vi "TestExec.Run Executable.vi"(6 "Reset":bool, 7 "Vars":variant, 8 "error in":errorcluster, 9 "Timeout(s)":dbl=500.0 caption="Time Out(s)" format="%.2f", 10 "Output Folder":path, 11 "Utility Config File":path) -> (0 "Error":errorcluster, 3 "RTN Data":T1 {"MeasData"."Status" items=["LOG", "PASS", "FAIL", "ERROR"]; "Attr"."Status" items=["LOG", "PASS", "FAIL", "ERROR"]; "Num"."Status" items=["LOG", "PASS", "FAIL", "ERROR"]})   [LabVIEW 2024]
uses:
  TestExec.Local Result Data.ctl
  Results/Result.Attribute.ctl
  Results/Result.Measurement and Attribute Item Status.ctl
  Results/Result.Numeric.ctl
  Results/Result.Limit Type.ctl
  Results/Result XML/TestResult.SW Item.ctl
  Reports/Report.Result FileDataObject.ctl
  Results/Result.Measurement Item.ctl
  Cmd Exe/CmdExe.Setup Params.ctl
  Cmd Exe/CmdExe.Output Error Check Setup.ctl
  <vilib>/Utility/error.llb/Trim Whitespace One-Sided.vi
  Errors.lvlib
  <vilib>/KATE/Time/Time Utils.lvlib
panel:
  in  "Tab Control":enum32{"Execute", "Results"}(tab)
  out "Active":bool
  out "Sys Exec Commands":string
  out "Sys Exec STDOut":string
  out "Dur(s)":dbl caption="Duration(s)" format="%.3f"
  out "Rslt":u32(colorbox)=13816530 caption="Exe"
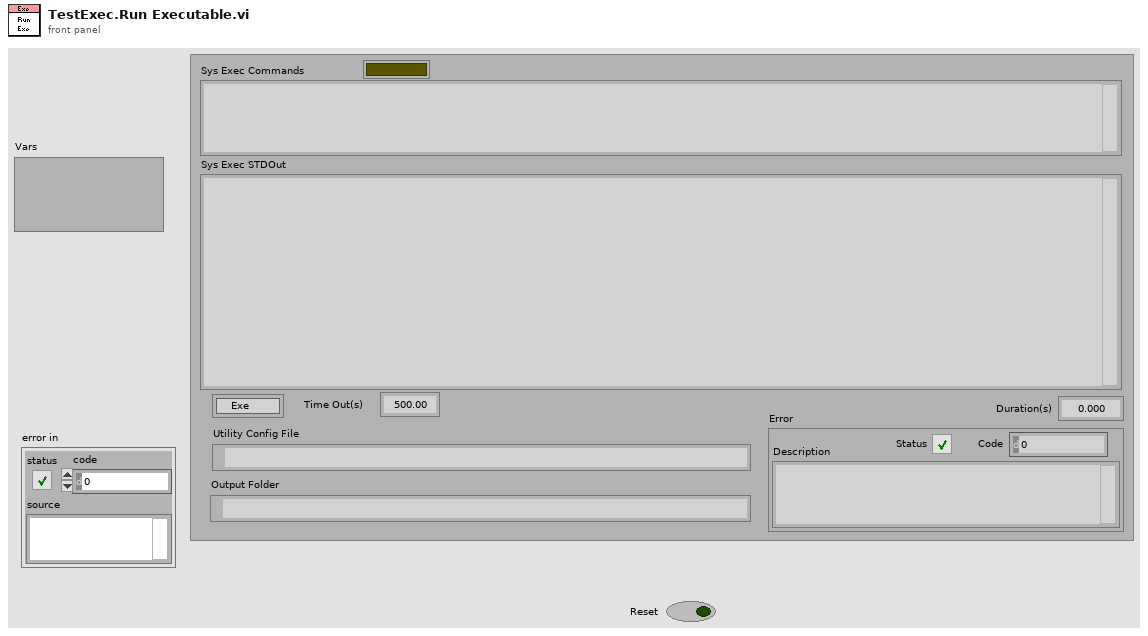
[diagram p1: front panel]
types:
  T1 = typedef "TestExec.Local Result Data.ctl" = cluster{"Attr":T2[], "Num":T4[], "UUT Props":string[][], "Vars":string[][], "SW Items":T6[], "Error":errorcluster, "Step":i32, "FileObjs":T7[], "MeasData":T8[]}
  T2 = typedef "Result.Attribute.ctl" = cluster{"Cnt":i32, "Step":string, "Category":string, "Name":string, "Value":string, "Status":T3, "Code":i32, "Desc":string, "Time":timestamp}
  T3 = typedef "Result.Measurement and Attribute Item Status.ctl" = i32
  T4 = typedef "Result.Numeric.ctl" = cluster{"Cnt":i32, "Step":string, "Category":string, "Name":string, "Value":dbl, "Units":string, "LimType":T5, "LL":dbl, "UL":dbl, "Status":T3, "Code":i32, "Desc":string, "Time":timestamp}
  T5 = typedef "Result.Limit Type.ctl" = enum16{"None", "EQ", "NE", "GT", "LT", "GE", "LE", "GTLT", "GELE", "GELT", "GTLE", "LTGT", "LEGE", "LEGT", "LTGE", "Contains", "NotContains"}
  T6 = typedef "TestResult.SW Item.ctl" = cluster{"Name":string, "PN":string, "Version":string, "Note":string}
  T7 = typedef "Report.Result FileDataObject.ctl" = cluster{"Cnt":i32, "Step":string, "Category":string, "Name":string, "Type":string, "File Name":string, "Time":string, "Path":path}
  T8 = typedef "Result.Measurement Item.ctl" = cluster{"Cnt":i32, "Step":string, "Category":string, "Name":string, "Value":string, "Units":string, "LimType":string, "LL":string, "UL":string, "Status":T3, "Code":i32, "Desc":string, "Time":timestamp}
  T9 = typedef "CmdExe.Setup Params.ctl" = cluster{"Timeout (s)":dbl, "Show Cmd Win":bool, "Error Check":T10, "Log_En":bool, "LogFileName":string, "LogDir":path}
  T10 = typedef "CmdExe.Output Error Check Setup.ctl" = cluster{"StdOut_Ck":bool, "StdOutErrMsgs":string[], "StdErr_Ck":bool, "RtnCode_Ck":bool, "RtnCodePASS":i32}
  T11 = cluster{"Args":string, "Setup":T9, "StdOut":string, "ActionName":string, "Exe":path, "RTN Data":T1, "Prefix":string, "Code":i32}
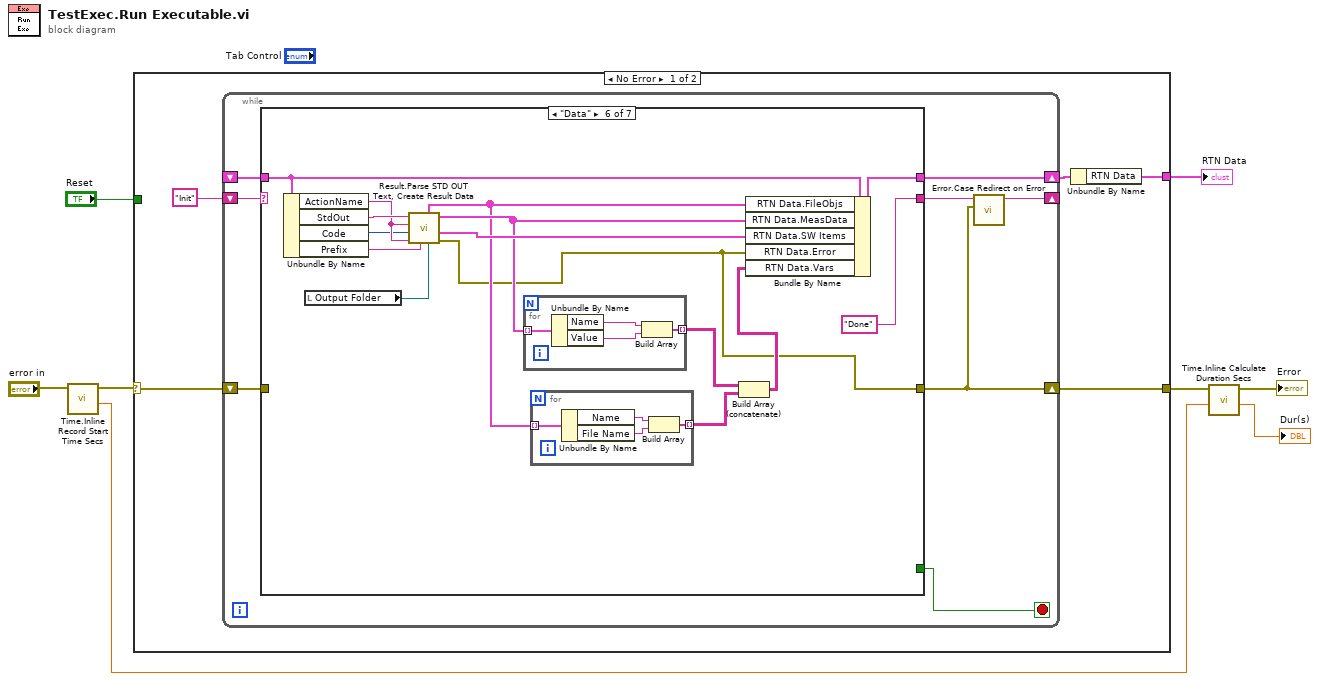
[diagram p0: block diagram]
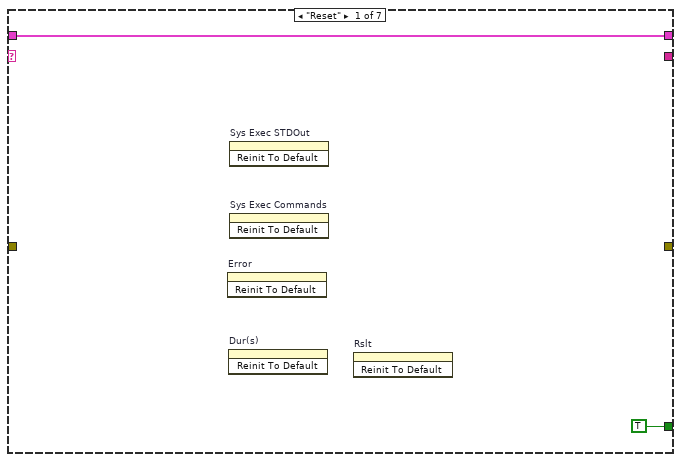
[diagram p2: hidden frame]
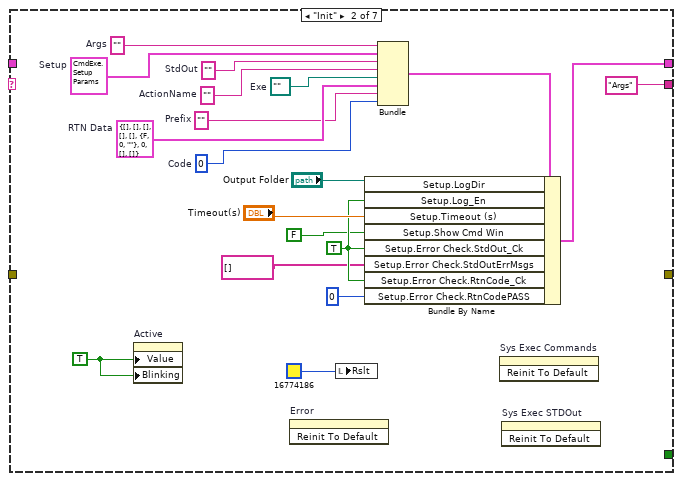
[diagram p3: hidden frame]
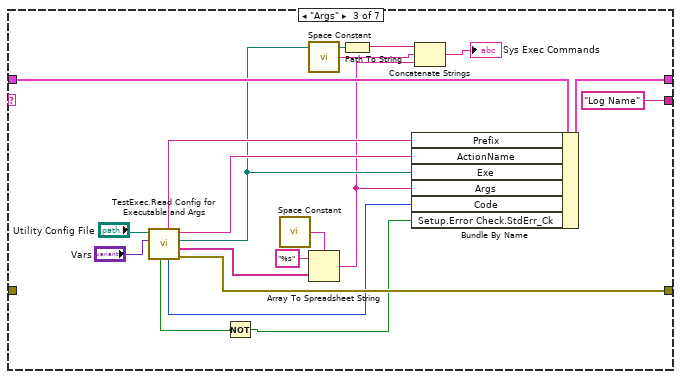
[diagram p4: hidden frame]
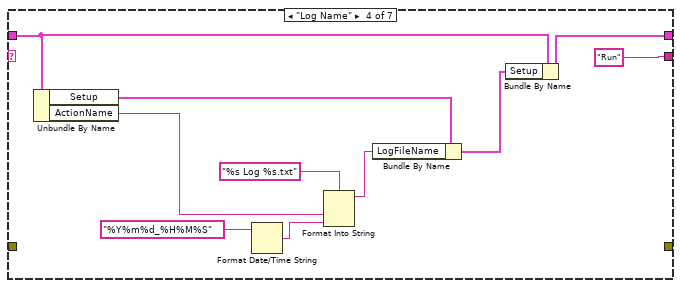
[diagram p5: hidden frame]
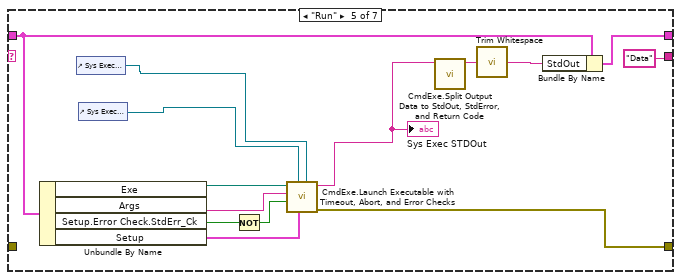
[diagram p6: hidden frame]
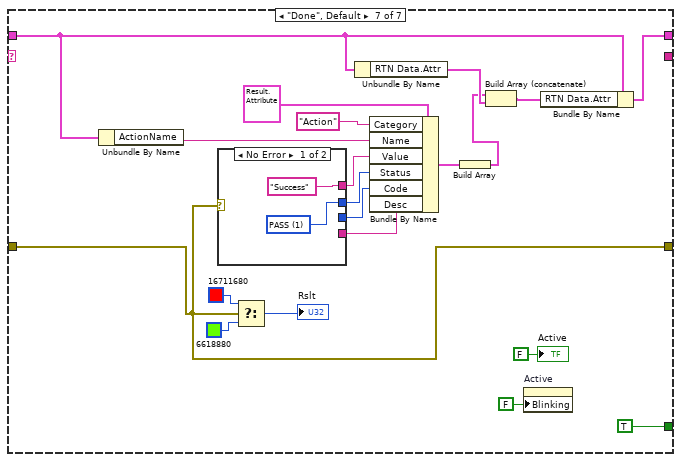
[diagram p7: hidden frame]
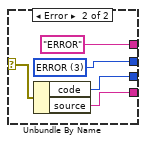
[diagram p8: hidden frame]
diagram:
  n1 = call <vilib>:"Time.Inline Record Start Time Secs.vi"("Error In Upper"="error in") -> ("Start(s)"=w2:dbl, "Error Out Upper"=w6:errorcluster)  [unwired: 8 in, 1 out]
  n2 = case shown="No Error" w6 {
    selector: w6 -> [w13 w136]
    tunnel: [w12 w136] -> w4
    tunnel: [w10 _] -> w8
    tunnel: "Reset" -> [_ _]
    frame No Error {
      n3 = while {
        shift-right: [w15] -> _
        shift-left: "Init" -> [w21]
        shift-right: [w20] -> w11
        shift-left: _ -> [w19]
        shift-right: [w14] -> w12
        shift-left: w13 -> [w17]
        stop <- w18 stop-if-true
        n4 = case shown="\"Data\"" w21 {
          tunnel: [_ "Args" "Log Name" "Run" "Data" "Done" _] -> w16
          tunnel: [w23 w34 w61 w70 w75 w97 w112] -> w20
          tunnel: w19 -> [w23 _ w60 w69 w77 w96 w111]
          tunnel: [TRUE _ _ _ _ _ TRUE] -> w18
          tunnel: w17 -> [_ _ _ _ _ _ w109]
          tunnel: [_ _ w53 _ w74 w88 w109] -> w14
          frame "Reset" {
            n5 = invoke on="Error" class="Clust (strict)" method="Reinit To Default"() -> ()  [unwired: 3 in, 3 out]
            n6 = invoke on="Dur(s)" class="DigNum (strict)" method="Reinit To Default"() -> ()  [unwired: 3 in, 3 out]
            n7 = invoke on="Sys Exec STDOut" class="Str" method="Reinit To Default"() -> ()  [unwired: 3 in, 3 out]
            n8 = invoke on="Sys Exec Commands" class="Str" method="Reinit To Default"() -> ()  [unwired: 3 in, 3 out]
            n9 = invoke on="Rslt" class="ColBox" method="Reinit To Default"() -> ()  [unwired: 3 in, 3 out]
          }
          frame "Init" {
            w24 = 0  # Code
            w25 = ""  # Prefix
            w26 = T1 {"Attr"=[], "Num"=[], "UUT Props"=[], "Vars"=[], "SW Items"=[], "Error"={"status"=FALSE, "code"=0, "source"=""}, "Step"=0, "FileObjs"=[], "MeasData"=[]}  # RTN Data
            w27 = path ""  # Exe
            w28 = ""  # ActionName
            w31 = ""  # StdOut
            w35 = TRUE
            w40 = TRUE ("Value")
            w39 = T9 {"Timeout (s)"=60.0, "Show Cmd Win"=FALSE, "Error Check"={"StdOut_Ck"=FALSE, "StdOutErrMsgs"=["Error", "Unable to find device "], "StdErr_Ck"=FALSE, "RtnCode_Ck"=FALSE, "RtnCodePASS"=0}, "Log_En"=FALSE, "LogFileName"="", "LogDir"=path ""}  # Setup
            w42 = ""  # Args
            n10 = property on="Active" class="Bool (strict)"("Value"=w40, "Blinking"=w40) -> ()  [unwired: 2 in, 2 out]
            n11 = invoke on="Error" class="Clust (strict)" method="Reinit To Default"() -> ()  [unwired: 3 in, 3 out]
            n12 = local write "Rslt"(u32 16774186) -> ()
            n13 = Bundle("Args"=w42, "Setup"=w39, "StdOut"=w31, "ActionName"=w28, "Exe"=w27, "RTN Data"=w26, "Prefix"=w25, "Code"=w24) -> (w36:T11)  [unwired: 1 in]
            n14 = Bundle By Name(cluster=w36, "Setup.LogDir"="Output Folder", "Setup.Log_En"=w35, "Setup.Timeout (s)"="Timeout(s)", "Setup.Show Cmd Win"=FALSE, "Setup.Error Check.StdOut_Ck"=w35, "Setup.Error Check.StdOutErrMsgs"=string[] [], "Setup.Error Check.RtnCode_Ck"=w35, "Setup.Error Check.RtnCodePASS"=0 ("Error Check.RtnCodePASS")) -> (w34:T11)
            n15 = invoke on="Sys Exec Commands" class="Str" method="Reinit To Default"() -> ()  [unwired: 3 in, 3 out]
            n16 = invoke on="Sys Exec STDOut" class="Str" method="Reinit To Default"() -> ()  [unwired: 3 in, 3 out]
          }
          frame "Args" {
            n17 = call "TestExec.Read Config for Executable and Args.vi"("Vars"="Vars", "Config File"="Utility Config File") -> ("error out"=w53:errorcluster, "Args"=w55:string[], "Exe"=w47:path, "Action Name"=w52:string, "Error Code"=w51:i32, "Data Name Prefix"=w50:string, "IgnoreStdError"=w44:bool)  [unwired: 2 in, 1 out]
            n18 = Not(x=w44) -> (.not. x?=w43:bool)
            n19 = call <vilib>:"Space Constant.vi"() -> ("String"=w56:string)
            n20 = call <vilib>:"Space Constant.vi"() -> ("String"=w45:string)
            n21 = Array To Spreadsheet String(delimiter (Tab)=w56, array=w55, 3:"%s" ("format string")) -> (spreadsheet string=w46:string)
            n22 = Path To String(path=w47) -> (string=w48:string)
            n23 = Bundle By Name(cluster=w60, "Prefix"=w50, "ActionName"=w52, "Exe"=w47, "Args"=w46, "Code"=w51, "Setup.Error Check.StdErr_Ck"=w43) -> (w61:T11)
            n24 = Concatenate Strings(w48, w45, w46) -> (→"Sys Exec Commands":string)
          }
          frame "Log Name" {
            n25 = Unbundle By Name(w69) -> ("Setup"=w67:T9, "ActionName"=w62:string)
            n26 = Format Date/Time String(time format string (%c)="%Y%m%d_%H%M%S") -> (date/time string=w63:string)  [unwired: 2 in]
            n27 = Format Into String(format string="%s Log %s.txt", w62, w63) -> (resulting string=w64:string)  [unwired: 2 in, 1 out]
            n28 = Bundle By Name(cluster=w67, "LogFileName"=w64) -> (w68:T9)
            n29 = Bundle By Name(cluster=w69, "Setup"=w68) -> (w70:T11)
          }
          frame "Run" {
            n30 = Unbundle By Name(w77) -> ("Exe"=w76:path, "Args"=w85:string, "Setup.Error Check.StdErr_Ck"=w73:bool, "Setup"=w84:T9)
            n31 = control-ref of="Sys Exec Commands"() -> (w83:refnum<vi>)
            n32 = control-ref of="Sys Exec STDOut"() -> (w82:refnum<vi>)
            n33 = Not(x=w73) -> (.not. x?=w72:bool)
            n34 = call "CmdExe.Launch Executable with Timeout, Abort, and Error Checks.vi"("Cmd IN Ref"=w83, "Setup"=w84, "Output Ref"=w82, "Ignore StdErr"=w72, "Args"=w85, "Executable"=w76) -> ("error out"=w74:errorcluster, "Data Out"=w79:string)  [unwired: 2 in, 2 out]
            "Sys Exec STDOut" <- w79
            n35 = call "CmdExe.Split Output Data to StdOut, StdError, and Return Code.vi"("Output Data"=w79) -> ("StdOut"=w80:string)  [unwired: 7 in, 3 out]
            n36 = call <vilib>:"Trim Whitespace.vi"("string"=w80) -> ("trimmed string"=w78:string)  [unwired: 1 in]
            n37 = Bundle By Name(cluster=w77, "StdOut"=w78) -> (w75:T11)
          }
          frame "Data" {
            n38 = Unbundle By Name(w96) -> ("ActionName"=w93:string, "StdOut"=w100:string, "Code"=w87:i32, "Prefix"=w86:string)
            n39 = local read "Output Folder"() -> (w98:path)
            n40 = call "Result.Parse STD OUT Text, Create Result Data.vi"("UUTDir"=w98, "Prefix"=w86, "Version Name"=w93, "Error Code"=w87, "Task Name"=w93, "StdOut"=w100) -> ("Error"=w88:errorcluster, "SW Ver"=w99:T6[], "Meas"=w95:T8[], "Data Files"=w94:T7[])  [unwired: 2 in]
            n41 = for {
              tunnel: w95 -> [w108] mode=indexing
              tunnel: [w105] -> w92 mode=indexing
              n42 = Unbundle By Name(w108) -> ("Name"=w107:string, "Value"=w106:string)
              n43 = Build Array(w107, w106) -> (w105:string[])
            }
            n44 = for {
              tunnel: w94 -> [w104] mode=indexing
              tunnel: [w102] -> w91 mode=indexing
              n45 = Unbundle By Name(w104) -> ("Name"=w103:string, "File Name"=w101:string)
              n46 = Build Array(w103, w101) -> (w102:string[])
            }
            n47 = Build Array (concatenate)(w92, w91) -> (w90:string[][])
            n48 = Bundle By Name(cluster=w96, "RTN Data.FileObjs"=w94, "RTN Data.MeasData"=w95, "RTN Data.SW Items"=w99, "RTN Data.Error"=w88, "RTN Data.Vars"=w90) -> (w97:T11)
          }
          frame "Done", Default {
            n49 = Unbundle By Name(w111) -> ("ActionName"=w110:string)
            n50 = case shown="No Error" w109 {
              selector: w109 -> [_ w134]
              tunnel: ["Success" "ERROR"] -> w122
              tunnel: [w130 w131] -> w119
              tunnel: [_ w133] -> w121
              tunnel: [_ w132] -> w120
              frame No Error {
                w130 = T3 1 items=["LOG", "PASS", "FAIL", "ERROR"] ("Status")
              }
              frame Error {
                w131 = T3 3 items=["LOG", "PASS", "FAIL", "ERROR"] ("Status")
                n51 = Unbundle By Name(w134) -> ("code"=w133:i32, "source"=w132:string)
              }
            }
            n52 = Select(t=u32 16711680, s=w109, f=u32 6618880) -> (s? t:f=→"Rslt":u32)
            n53 = Unbundle By Name(w111) -> ("RTN Data.Attr"=w115:T2[])
            n54 = Bundle By Name(cluster=T2 {"Cnt"=0, "Step"="", "Category"="", "Name"="", "Value"="", "Status"=0, "Code"=0, "Desc"="", "Time"=timestamp(0 s since 1904-01-01)} ("Attribute"), "Category"="Action", "Name"=w110, "Value"=w122, "Status"=w119, "Code"=w121, "Desc"=w120) -> (w117:T2)
            n55 = Build Array(w117) -> (w114:T2[])
            n56 = Build Array (concatenate)(w114, w115) -> (w116:T2[])
            n57 = property on="Active" class="Bool (strict)"("Blinking"=FALSE ("Value")) -> ()  [unwired: 2 in, 2 out]
            n58 = Bundle By Name(cluster=w111, "RTN Data.Attr"=w116) -> (w112:T11)
            "Active" <- FALSE ("Active")
          }
        }
        n59 = call "Error.Case Redirect on Error.vi"("error in"=w14, "Next Case"=w16) -> ("Next Case Out"=w15:string)  [unwired: 9 in]
      }
      n60 = Unbundle By Name(w11) -> ("RTN Data"=w10:T1)
    }
    frame Error {
    }
  }
  "RTN Data" <- w8
  n61 = call <vilib>:"Time.Inline Calculate Duration Secs.vi"("Start(Sec)"=w2, "Error In Top"=w4) -> ("Duration(s)"=→"Dur(s)":dbl, "Error Out Top"=→"Error":errorcluster)  [unwired: 7 in, 1 out]
